vi "Save Intensity Dep Data.vi"(0 "Experiment Indicator":string, 1 "No. of Suns":dbl, 2 "Date array":string[](array[string]), 3 "Scan direction":i32, 4 "Data Array":dbl[][](array[numeric]), 6 "Username":string, 7 "Stabilisation time (ms)":dbl, 8 "Cell details cluster":T1={"Cell Position"=16, "Cell Label"="", "Pixel to measure"=0, "Area (cm^2)"=0.126, "Variable"="", "Variable value"="", "Scan settings in queue"=0, "Light or dark"="", "Measurement Type"=""} {"Pixel to measure" items=["All", "1", "2", "3", "4", "5", "6", "7", "8"]}, 10 "Measurement Delay (ms)":dbl=1.0, 11 "Stabilisation level \n(A or V depending on mode)":dbl=-1.4, 13 "Stabilisation Data":dbl[][](array[numeric])) -> (14 "Master Log":string[][](table), 15 "File path for master log":path, 17 "File path for JV data":path, 18 "File path for JV image":path)   [LabVIEW 2016]
uses:
  <vilib>/Utility/file.llb/Write To Spreadsheet File (string).vi
  <vilib>/Utility/file.llb/Read From Spreadsheet File (string).vi
  <vilib>/Analysis/NI_AALPro.lvlib
panel:
  in  "Scan rate (V/s)":dbl
  out "Vmp":dbl
  out "PCE":dbl
  out "FF":dbl
  out "Voc":dbl
  out "Jsc":dbl
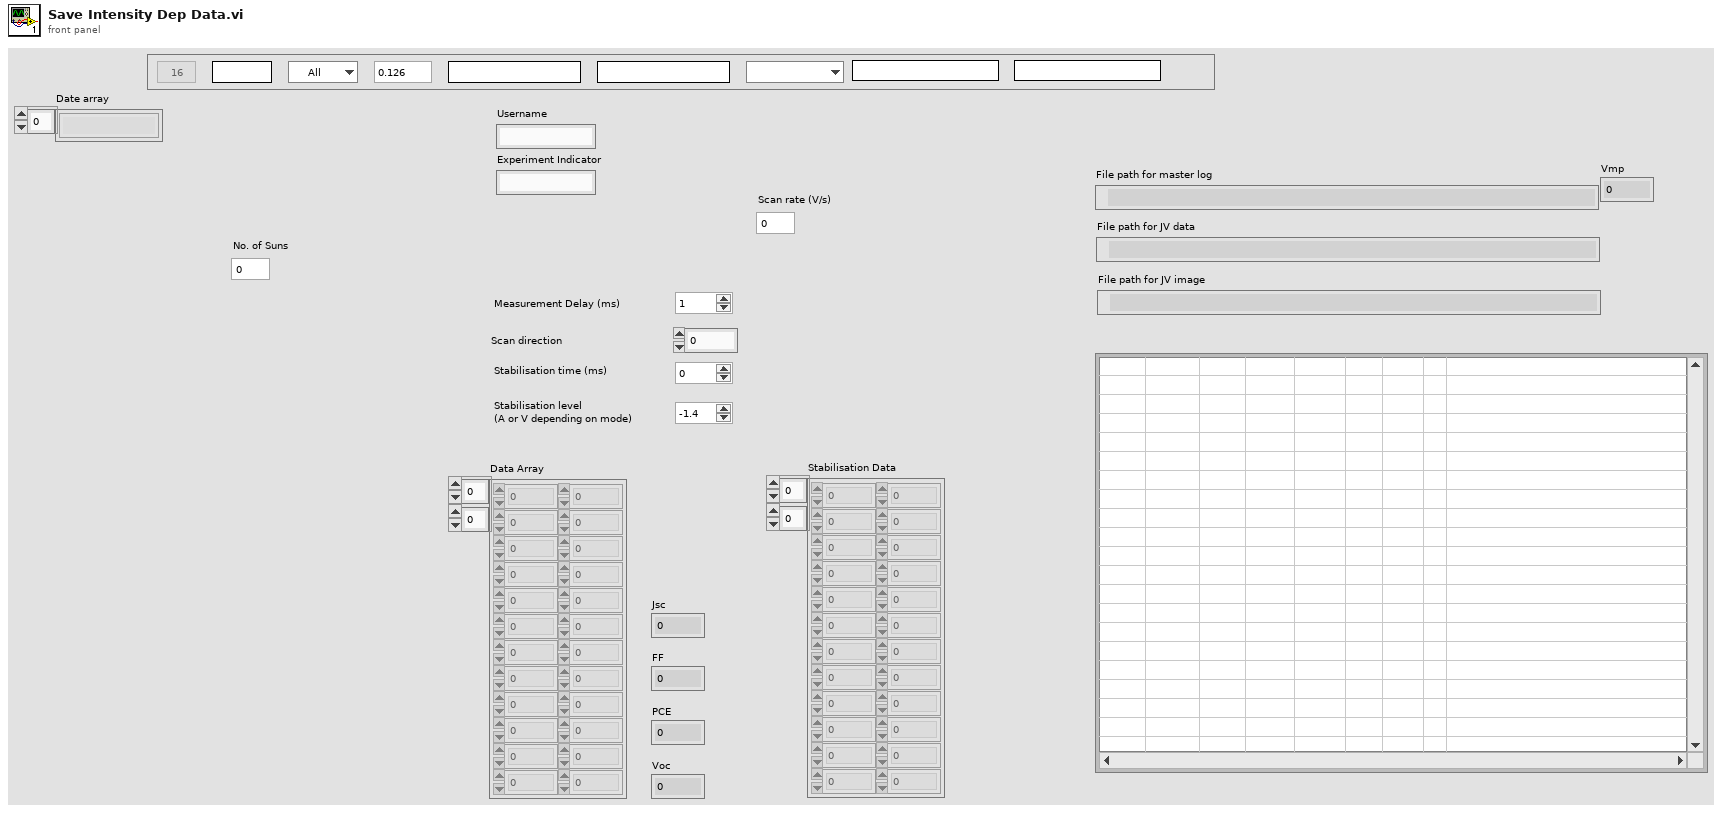
[diagram p1: front panel]
types:
  T1 = cluster{"Cell Position":i32, "Cell Label":string, "Pixel to measure":u16, "Area (cm^2)":dbl, "Variable":string, "Variable value":string, "Scan settings in queue":u16, "Light or dark":string, "Measurement Type":string}
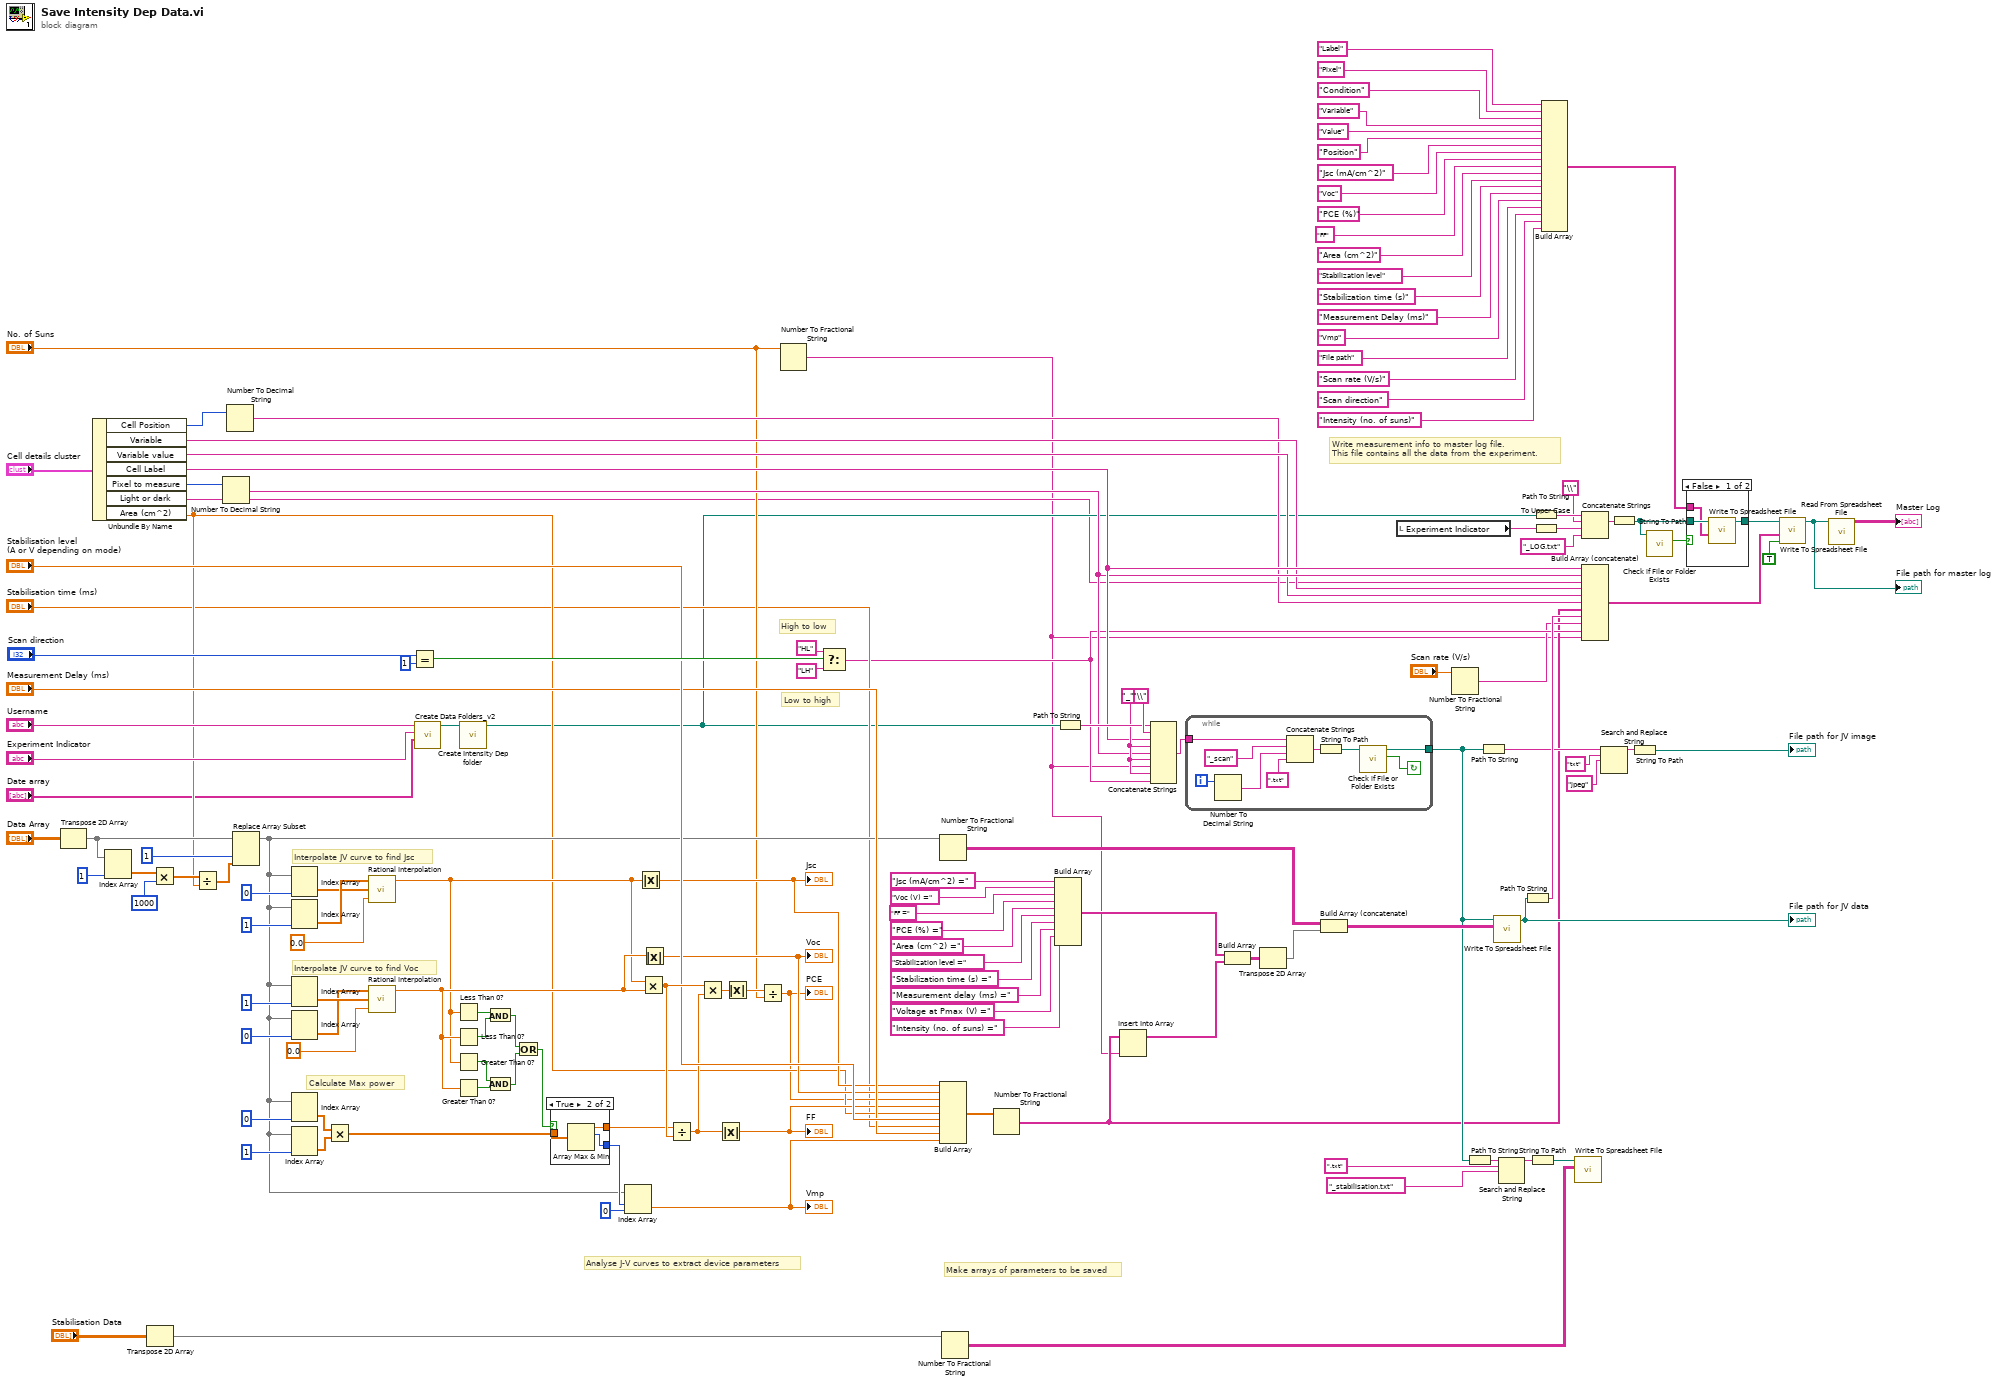
[diagram p0: block diagram]
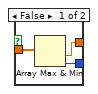
[diagram p3: hidden frame]
diagram:
  w62 = "_"
  # "Make arrays of parameters to be saved"
  # "Calculate Max power"
  # "Interpolate JV curve to find Voc"
  # "Interpolate JV curve to find Jsc"
  # "Analyse J-V curves to extract device parameters"
  # "Write measurement info to master log file.\nThis file contains all the data from the experiment."
  # "Low to high"
  # "High to low"
  n1 = Transpose 2D Array(2D array="Data Array") -> (transposed array=w70:dbl[][])
  n2 = Unbundle By Name("Cell details cluster") -> ("Cell Position"=w44:i32, "Variable"=w41:string, "Variable value"=w40:string, "Cell Label"=w43:string, "Pixel to measure"=w45:u16, "Light or dark"=w9:string, "Area (cm^2)"=w46:dbl)
  n3 = Index Array(array=w70, index (col)=1) -> (element=w68:dbl[])  [unwired: 1 in]
  n4 = Transpose 2D Array(2D array="Stabilisation Data") -> (transposed array=w53:dbl[][])
  n5 = Multiply(x=w68, y=1000) -> (x*y=w65:dbl[])
  n6 = Divide(x=w65, y=w46) -> (x/y=w64:dbl[])
  n7 = Number To Decimal String(number=w45) -> (decimal integer string=w42:string)  [unwired: 1 in]
  n8 = Number To Decimal String(number=w44) -> (decimal integer string=w39:string)  [unwired: 1 in]
  n9 = Replace Array Subset(array=w70, new element=w64, index (col)=1) -> (w50:dbl[][])  [unwired: 1 in]
  n10 = Index Array(array=w50, index (col)=0) -> (element=w133:dbl[])  [unwired: 1 in]
  n11 = Index Array(array=w50, index (col)=1) -> (element=w134:dbl[])  [unwired: 1 in]
  n12 = Index Array(array=w50, index (col)=1) -> (element=w132:dbl[])  [unwired: 1 in]
  n13 = Index Array(array=w50, index (col)=0) -> (element=w130:dbl[])  [unwired: 1 in]
  n14 = Index Array(array=w50, index (col)=0) -> (element=w138:dbl[])  [unwired: 1 in]
  n15 = Index Array(array=w50, index (col)=1) -> (element=w137:dbl[])  [unwired: 1 in]
  n16 = Multiply(x=w138, y=w137) -> (x*y=w131:dbl[])
  n17 = call <vilib>:"Rational Interpolation.vi"("x value"=0.0, "X"=w133, "Y"=w134) -> ("interpolation value"=w66:dbl)  [unwired: 2 out]
  n18 = call <vilib>:"Rational Interpolation.vi"("x value"=0.0, "X"=w132, "Y"=w130) -> ("interpolation value"=w76:dbl)  [unwired: 2 out]
  n19 = Equal?(x="Scan direction", y=1) -> (x = y?=w97:bool)
  n20 = call "Create Data Folders_v2.vi"("Date array"="Date array", "Experiment Indicator"="Experiment Indicator", "username"="Username") -> ("Data Output Folder"=w17:path)  [unwired: 8 in]
  n21 = Less Than 0?(x=w66) -> (x < 0?=w82:bool)
  n22 = Less Than 0?(x=w76) -> (x < 0?=w79:bool)
  n23 = Greater Than 0?(x=w66) -> (x > 0?=w80:bool)
  n24 = Greater Than 0?(x=w76) -> (x > 0?=w81:bool)
  n25 = call "Create Intensity Dep folder.vi"("Data Folder In"=w17) -> ("Data Output Folder"=w16:path)  [unwired: 10 in]
  n26 = And(x=w82, y=w79) -> (x .and. y?=w84:bool)
  n27 = And(x=w80, y=w81) -> (x .and. y?=w83:bool)
  n28 = Or(x=w84, y=w83) -> (x .or. y?=w78:bool)
  n29 = case shown="True" w78 {
    tunnel: [w146 w150] -> w63
    tunnel: w131 -> [w147 w149]
    tunnel: [w145 w148] -> w51
    frame False {
      n30 = Array Max & Min(array=w147) -> (min value=w146:dbl, min index (indices)=w145:i32)  [unwired: 2 out]
    }
    frame True {
      n31 = Array Max & Min(array=w149) -> (max value=w150:dbl, max index (indices)=w148:i32)  [unwired: 2 out]
    }
  }
  n32 = Index Array(array=w50, index (row)=w51, index (col)=0) -> (element=w48:dbl)
  "Vmp" <- w48
  n33 = Absolute Value(x=w66) -> (abs(x)=w77:dbl)
  "Jsc" <- w77
  n34 = Multiply(x=w66, y=w76) -> (x*y=w129:dbl)
  n35 = Absolute Value(x=w76) -> (abs(x)=w75:dbl)
  "Voc" <- w75
  n36 = Divide(x=w63, y=w129) -> (x/y=w73:dbl)
  n37 = Multiply(x=w129, y=w73) -> (x*y=w74:dbl)
  n38 = Absolute Value(x=w73) -> (abs(x)=w72:dbl)
  "FF" <- w72
  n39 = Absolute Value(x=w74) -> (abs(x)=w20:dbl)
  n40 = Divide(x=w20, y="No. of Suns") -> (x/y=w21:dbl)
  "PCE" <- w21
  n41 = Number To Fractional String(number="No. of Suns") -> (F-format string=w2:string)  [unwired: 3 in]
  n42 = Select(t="HL", s=w97, f="LH") -> (s? t:f=w8:string)
  n43 = Number To Fractional String(number=w50) -> (F-format string=w99:string[][])  [unwired: 3 in]
  n44 = Build Array(w77, w75, w21, w72, w46, "Stabilisation level \n(A or V depending on mode)", "Stabilisation time (ms)", "Measurement Delay (ms)", w48) -> (w124:dbl[])
  n45 = Number To Fractional String(number=w53) -> (F-format string=w54:string[][])  [unwired: 3 in]
  n46 = Number To Fractional String(number=w124) -> (F-format string=w4:string[])  [unwired: 3 in]
  n47 = Build Array("Jsc (mA/cm^2) =", "Voc (V) =", "FF =", "PCE (%) =", "Area (cm^2) =", "Stabilization level =", "Stabilization time (s) =", "Measurement delay (ms) =", "Voltage at Pmax (V) =", "Intensity (no. of suns) =") -> (w123:string[])
  n48 = Path To String(path=w16) -> (string=w108:string)
  n49 = Insert Into Array(array=w4, new element=w2) -> (w3:string[])  [unwired: 1 in]
  n50 = Concatenate Strings(w108, "\\", w43, w62, w42, w62, w2, w62, w8) -> (w89:string)
  n51 = while {
    tunnel: w89 -> [w159]
    tunnel: [w151] -> w60
    i -> [w157]
    stop <- w152 continue-if-true
    n52 = Number To Decimal String(number=w157) -> (decimal integer string=w156:string)  [unwired: 1 in]
    n53 = Concatenate Strings(w159, "_scan", w156, ".txt") -> (w153:string)
    n54 = String To Path(string=w153) -> (path=w154:path)
    n55 = call <vilib>:"Check if File or Folder Exists.vi"("path"=w154) -> ("file or folder exists?"=w152:bool, "dup path"=w151:path)  [unwired: 8 in, 1 out]
  }
  n56 = Build Array(w123, w3) -> (w119:string[][])
  n57 = Transpose 2D Array(2D array=w119) -> (transposed array=w118:string[][])
  n58 = Build Array (concatenate)(w99, w118) -> (w122:string[][])
  n59 = local read "Experiment Indicator"() -> (w85:string)
  n60 = Number To Fractional String(number="Scan rate (V/s)") -> (F-format string=w6:string)  [unwired: 3 in]
  n61 = Path To String(path=w60) -> (string=w59:string)
  n62 = Path To String(path=w60) -> (string=w88:string)
  n63 = call-poly <vilib>:"Write To Spreadsheet File.vi"("2D data"=w122, "file path (dialog if empty)"=w60) -> ("new file path (Not A Path if cancelled)"=w95:path)  [unwired: 6 in]
  "File path for JV data" <- w95
  n64 = Search and Replace String(input string=w59, search string=".txt", replace string="_stabilisation.txt") -> (result string=w56:string)  [unwired: 5 in, 3 out]
  n65 = Path To String(path=w95) -> (string=w90:string)
  n66 = String To Path(string=w56) -> (path=w55:path)
  n67 = Path To String(path=w16) -> (string=w114:string)
  n68 = To Upper Case(1:w85) -> (0:w86:string)
  n69 = Build Array("Label", "Pixel", "Condition", "Variable", "Value", "Position", "Jsc (mA/cm^2)", "Voc", "PCE (%)", "FF", "Area (cm^2)", "Stabilization level", "Stabilization time (s)", "Measurement Delay (ms)", "Vmp", "File path", "Scan rate (V/s)", "Scan direction", "Intensity (no. of suns)") -> (w22:string[])
  n70 = call-poly <vilib>:"Write To Spreadsheet File.vi"("2D data"=w54, "file path (dialog if empty)"=w55) -> ()  [unwired: 6 in, 1 out]
  n71 = Concatenate Strings(w114, "\\", w86, "_LOG.txt") -> (w112:string)
  n72 = Build Array (concatenate)(w43, w42, w9, w41, w40, w39, w4, w90, w6, w8, w2) -> (w111:string[])
  n73 = Search and Replace String(input string=w88, search string="txt", replace string="jpeg") -> (result string=w107:string)  [unwired: 5 in, 3 out]
  n74 = String To Path(string=w112) -> (path=w24:path)
  n75 = String To Path(string=w107) -> (path=→"File path for JV image":path)
  n76 = call <vilib>:"Check if File or Folder Exists.vi"("path"=w24) -> ("file or folder exists?"=w25:bool)  [unwired: 8 in, 2 out]
  n77 = case shown="False" w25 {
    tunnel: w24 -> [w162 w163]
    tunnel: [w161 w163] -> w23
    tunnel: w22 -> [w160 _]
    frame False {
      n78 = call-poly <vilib>:"Write To Spreadsheet File.vi"("1D data"=w160, "file path (dialog if empty)"=w162) -> ("new file path (Not A Path if cancelled)"=w161:path)  [unwired: 6 in]
    }
    frame True {
    }
  }
  n79 = call-poly <vilib>:"Write To Spreadsheet File.vi"("append to file? (new file:F)"=TRUE, "1D data"=w111, "file path (dialog if empty)"=w23) -> ("new file path (Not A Path if cancelled)"=w102:path)  [unwired: 5 in]
  "File path for master log" <- w102
  n80 = call-poly <vilib>:"Read From Spreadsheet File.vi"("file path (dialog if empty)"=w102) -> ("all rows"=→"Master Log":string[][])  [unwired: 6 in, 4 out]
